vi "App - analyze RUS V6.vi"() -> ()   [LabVIEW 2018] (continued)
__130814c/5_Cooling_2nd_try/September_2014/091714/83.49500K_500_2500_2.10000V_0.00000T_Sep17-2014__00-50-47_001_091714.bin", "last mod"=timestamp(3493774247 s since 1904-01-01), "file name str"="D:\\Data\\Ultrasound\\LSCO\\LSCO22__130814c\\5_Cooling_2nd_try\\September_2014\\091714\\83.49500K_500_2500_2.10000V_0.00000T_Sep17-2014__00-50-47_001_091714.bin", "mod time(min)"=58229570.78333333, "file format"=enum."binary", "power(V)"=2.1, "Magn Field(T) "=0.0}, {"temperature"=83.396, "temperature str"="83.39600", "file path"=path "D:/Data/Ultrasound/LSCO/LSCO22__130814c/5_Cooling_2nd_try/September_2014/091714/83.39600K_500_2500_2.10000V_0.00000T_Sep17-2014__00-52-06_001_091714.bin", "last mod"=timestamp(3493774326 s since 1904-01-01), "file name str"="D:\\Data\\Ultrasound\\LSCO\\LSCO22__130814c\\5_Cooling_2nd_try\\September_2014\\091714\\83.39600K_500_2500_2.10000V_0.00000T_Sep17-2014__00-52-06_001_091714.bin", "mod time(min)"=58229572.1, "file format"=enum."binary", "power(V)"=2.1, "Magn Field(T) "=0.0}, {"temperature"=83.298, "temperature str"="83.29800", "file path"=path "D:/Data/Ultrasound/LSCO/LSCO22__130814c/5_Cooling_2nd_try/September_2014/091714/83.29800K_500_2500_2.10000V_0.00000T_Sep17-2014__00-53-26_001_091714.bin", "last mod"=timestamp(3493774406 s since 1904-01-01), "file name str"="D:\\Data\\Ultrasound\\LSCO\\LSCO22__130814c\\5_Cooling_2nd_try\\September_2014\\091714\\83.29800K_500_2500_2.10000V_0.00000T_Sep17-2014__00-53-26_001_091714.bin", "mod time(min)"=58229573.43333333, "file format"=enum."binary", "power(V)"=2.1, "Magn Field(T) "=0.0}, {"temperature"=83.202, "temperature str"="83.20200", "file path"=path "D:/Data/Ultrasound/LSCO/LSCO22__130814c/5_Cooling_2nd_try/September_2014/091714/83.20200K_500_2500_2.10000V_0.00000T_Sep17-2014__00-54-45_001_091714.bin", "last mod"=timestamp(3493774485 s since 1904-01-01), "file name str"="D:\\Data\\Ultrasound\\LSCO\\LSCO22__130814c\\5_Cooling_2nd_try\\September_2014\\091714\\83.20200K_500_2500_2.10000V_0.00000T_Sep17-2014__00-54-45_001_091714.bin", "mod time(min)"=58229574.75, "file format"=enum."binary", "power(V)"=2.1, "Magn Field(T) "=0.0}, {"temperature"=83.102, "temperature str"="83.10200", "file path"=path "D:/Data/Ultrasound/LSCO/LSCO22__130814c/5_Cooling_2nd_try/September_2014/091714/83.10200K_500_2500_2.10000V_0.00000T_Sep17-2014__00-56-04_001_091714.bin", "last mod"=timestamp(3493774564 s since 1904-01-01), "file name str"="D:\\Data\\Ultrasound\\LSCO\\LSCO22__130814c\\5_Cooling_2nd_try\\September_2014\\091714\\83.10200K_500_2500_2.10000V_0.00000T_Sep17-2014__00-56-04_001_091714.bin", "mod time(min)"=58229576.06666667, "file format"=enum."binary", "power(V)"=2.1, "Magn Field(T) "=0.0}, {"temperature"=83.008, "temperature str"="83.00800", "file path"=path "D:/Data/Ultrasound/LSCO/LSCO22__130814c/5_Cooling_2nd_try/September_2014/091714/83.00800K_500_2500_2.10000V_0.00000T_Sep17-2014__00-57-24_001_091714.bin", "last mod"=timestamp(3493774644 s since 1904-01-01), "file name str"="D:\\Data\\Ultrasound\\LSCO\\LSCO22__130814c\\5_Cooling_2nd_try\\September_2014\\091714\\83.00800K_500_2500_2.10000V_0.00000T_Sep17-2014__00-57-24_001_091714.bin", "mod time(min)"=58229577.4, "file format"=enum."binary", "power(V)"=2.1, "Magn Field(T) "=0.0}, {"temperature"=82.91, "temperature str"="82.91000", "file path"=path "D:/Data/Ultrasound/LSCO/LSCO22__130814c/5_Cooling_2nd_try/September_2014/091714/82.91000K_500_2500_2.10000V_0.00000T_Sep17-2014__00-58-43_001_091714.bin", "last mod"=timestamp(3493774723 s since 1904-01-01), "file name str"="D:\\Data\\Ultrasound\\LSCO\\LSCO22__130814c\\5_Cooling_2nd_try\\September_2014\\091714\\82.91000K_500_2500_2.10000V_0.00000T_Sep17-2014__00-58-43_001_091714.bin", "mod time(min)"=58229578.71666667, "file format"=enum."binary", "power(V)"=2.1, "Magn Field(T) "=0.0}, {"temperature"=82.813, "temperature str"="82.81300", "file path"=path "D:/Data/Ultrasound/LSCO/LSCO22__130814c/5_Cooling_2nd_try/September_2014/091714/82.81300K_500_2500_2.10000V_0.00000T_Sep17-2014__01-00-03_001_091714.bin", "last mod"=timestamp(3493774803 s since 1904-01-01), "file name str"="D:\\Data\\Ultrasound\\LSCO\\LSCO22__130814c\\5_Cooling_2nd_try\\September_2014\\091714\\82.81300K_500_2500_2.10000V_0.00000T_Sep17-2014__01-00-03_001_091714.bin", "mod time(min)"=58229580.05, "file format"=enum."binary", "power(V)"=2.1, "Magn Field(T) "=0.0}, {"temperature"=82.719, "temperature str"="82.71900", "file path"=path "D:/Data/Ultrasound/LSCO/LSCO22__130814c/5_Cooling_2nd_try/September_2014/091714/82.71900K_500_2500_2.10000V_0.00000T_Sep17-2014__01-01-22_001_091714.bin", "last mod"=timestamp(3493774882 s since 1904-01-01), "file name str"="D:\\Data\\Ultrasound\\LSCO\\LSCO22__130814c\\5_Cooling_2nd_try\\September_2014\\091714\\82.71900K_500_2500_2.10000V_0.00000T_Sep17-2014__01-01-22_001_091714.bin", "mod time(min)"=58229581.36666667, "file format"=enum."binary", "power(V)"=2.1, "Magn Field(T) "=0.0}, {"temperature"=82.621, "temperature str"="82.62100", "file path"=path "D:/Data/Ultrasound/LSCO/LSCO22__130814c/5_Cooling_2nd_try/September_2014/091714/82.62100K_500_2500_2.10000V_0.00000T_Sep17-2014__01-02-41_001_091714.bin", "last mod"=timestamp(3493774961 s since 1904-01-01), "file name str"="D:\\Data\\Ultrasound\\LSCO\\LSCO22__130814c\\5_Cooling_2nd_try\\September_2014\\091714\\82.62100K_500_2500_2.10000V_0.00000T_Sep17-2014__01-02-41_001_091714.bin", "mod time(min)"=58229582.68333333, "file format"=enum."binary", "power(V)"=2.1, "Magn Field(T) "=0.0}, {"temperature"=82.529, "temperature str"="82.52900", "file path"=path "D:/Data/Ultrasound/LSCO/LSCO22__130814c/5_Cooling_2nd_try/September_2014/091714/82.52900K_500_2500_2.10000V_0.00000T_Sep17-2014__01-04-01_001_091714.bin", "last mod"=timestamp(3493775041 s since 1904-01-01), "file name str"="D:\\Data\\Ultrasound\\LSCO\\LSCO22__130814c\\5_Cooling_2nd_try\\September_2014\\091714\\82.52900K_500_2500_2.10000V_0.00000T_Sep17-2014__01-04-01_001_091714.bin", "mod time(min)"=58229584.016666666, "file format"=enum."binary", "power(V)"=2.1, "Magn Field(T) "=0.0}, {"temperature"=82.431, "temperature str"="82.43100", "file path"=path "D:/Data/Ultrasound/LSCO/LSCO22__130814c/5_Cooling_2nd_try/September_2014/091714/82.43100K_500_2500_2.10000V_0.00000T_Sep17-2014__01-05-20_001_091714.bin", "last mod"=timestamp(3493775120 s since 1904-01-01), "file name str"="D:\\Data\\Ultrasound\\LSCO\\LSCO22__130814c\\5_Cooling_2nd_try\\September_2014\\091714\\82.43100K_500_2500_2.10000V_0.00000T_Sep17-2014__01-05-20_001_091714.bin", "mod time(min)"=58229585.333333336, "file format"=enum."binary", "power(V)"=2.1, "Magn Field(T) "=0.0}, {"temperature"=82.336, "temperature str"="82.33600", "file path"=path "D:/Data/Ultrasound/LSCO/LSCO22__130814c/5_Cooling_2nd_try/September_2014/091714/82.33600K_500_2500_2.10000V_0.00000T_Sep17-2014__01-06-40_001_091714.bin", "last mod"=timestamp(3493775200 s since 1904-01-01), "file name str"="D:\\Data\\Ultrasound\\LSCO\\LSCO22__130814c\\5_Cooling_2nd_try\\September_2014\\091714\\82.33600K_500_2500_2.10000V_0.00000T_Sep17-2014__01-06-40_001_091714.bin", "mod time(min)"=58229586.666666664, "file format"=enum."binary", "power(V)"=2.1, "Magn Field(T) "=0.0}, {"temperature"=82.244, "temperature str"="82.24400", "file path"=path "D:/Data/Ultrasound/LSCO/LSCO22__130814c/5_Cooling_2nd_try/September_2014/091714/82.24400K_500_2500_2.10000V_0.00000T_Sep17-2014__01-07-59_001_091714.bin", "last mod"=timestamp(3493775279 s since 1904-01-01), "file name str"="D:\\Data\\Ultrasound\\LSCO\\LSCO22__130814c\\5_Cooling_2nd_try\\September_2014\\091714\\82.24400K_500_2500_2.10000V_0.00000T_Sep17-2014__01-07-59_001_091714.bin", "mod time(min)"=58229587.983333334, "file format"=enum."binary", "power(V)"=2.1, "Magn Field(T) "=0.0}, {"temperature"=82.149, "temperature str"="82.14900", "file path"=path "D:/Data/Ultrasound/LSCO/LSCO22__130814c/5_Cooling_2nd_try/September_2014/091714/82.14900K_500_2500_2.10000V_0.00000T_Sep17-2014__01-09-19_001_091714.bin", "last mod"=timestamp(3493775359 s since 1904-01-01), "file name str"="D:\\Data\\Ultrasound\\LSCO\\LSCO22__130814c\\5_Cooling_2nd_try\\September_2014\\091714\\82.14900K_500_2500_2.10000V_0.00000T_Sep17-2014__01-09-19_001_091714.bin", "mod time(min)"=58229589.31666667, "file format"=enum."binary", "power(V)"=2.1, "Magn Field(T) "=0.0}, {"temperature"=82.054, "temperature str"="82.05400", "file path"=path "D:/Data/Ultrasound/LSCO/LSCO22__130814c/5_Cooling_2nd_try/September_2014/091714/82.05400K_500_2500_2.10000V_0.00000T_Sep17-2014__01-10-38_001_091714.bin", "last mod"=timestamp(3493775438 s since 1904-01-01), "file name str"="D:\\Data\\Ultrasound\\LSCO\\LSCO22__130814c\\5_Cooling_2nd_try\\September_2014\\091714\\82.05400K_500_2500_2.10000V_0.00000T_Sep17-2014__01-10-38_001_091714.bin", "mod time(min)"=58229590.63333333, "file format"=enum."binary", "power(V)"=2.1, "Magn Field(T) "=0.0}, {"temperature"=81.963, "temperature str"="81.96300", "file path"=path "D:/Data/Ultrasound/LSCO/LSCO22__130814c/5_Cooling_2nd_try/September_2014/091714/81.96300K_500_2500_2.10000V_0.00000T_Sep17-2014__01-11-58_001_091714.bin", "last mod"=timestamp(3493775518 s since 1904-01-01), "file name str"="D:\\Data\\Ultrasound\\LSCO\\LSCO22__130814c\\5_Cooling_2nd_try\\September_2014\\091714\\81.96300K_500_2500_2.10000V_0.00000T_Sep17-2014__01-11-58_001_091714.bin", "mod time(min)"=58229591.96666667, "file format"=enum."binary", "power(V)"=2.1, "Magn Field(T) "=0.0}, {"temperature"=81.869, "temperature str"="81.86900", "file path"=path "D:/Data/Ultrasound/LSCO/LSCO22__130814c/5_Cooling_2nd_try/September_2014/091714/81.86900K_500_2500_2.10000V_0.00000T_Sep17-2014__01-13-17_001_091714.bin", "last mod"=timestamp(3493775597 s since 1904-01-01), "file name str"="D:\\Data\\Ultrasound\\LSCO\\LSCO22__130814c\\5_Cooling_2nd_try\\September_2014\\091714\\81.86900K_500_2500_2.10000V_0.00000T_Sep17-2014__01-13-17_001_091714.bin", "mod time(min)"=58229593.28333333, "file format"=enum."binary", "power(V)"=2.1, "Magn Field(T) "=0.0}, {"temperature"=81.779, "temperature str"="81.77900", "file path"=path "D:/Data/Ultrasound/LSCO/LSCO22__130814c/5_Cooling_2nd_try/September_2014/091714/81.77900K_500_2500_2.10000V_0.00000T_Sep17-2014__01-14-37_001_091714.bin", "last mod"=timestamp(3493775677 s since 1904-01-01), "file name str"="D:\\Data\\Ultrasound\\LSCO\\LSCO22__130814c\\5_Cooling_2nd_try\\September_2014\\091714\\81.77900K_500_2500_2.10000V_0.00000T_Sep17-2014__01-14-37_001_091714.bin", "mod time(min)"=58229594.61666667, "file format"=enum."binary", "power(V)"=2.1, "Magn Field(T) "=0.0}, {"temperature"=81.683, "temperature str"="81.68300", "file path"=path "D:/Data/Ultrasound/LSCO/LSCO22__130814c/5_Cooling_2nd_try/September_2014/091714/81.68300K_500_2500_2.10000V_0.00000T_Sep17-2014__01-15-56_001_091714.bin", "last mod"=timestamp(3493775756 s since 1904-01-01), "file name str"="D:\\Data\\Ultrasound\\LSCO\\LSCO22__130814c\\5_Cooling_2nd_try\\September_2014\\091714\\81.68300K_500_2500_2.10000V_0.00000T_Sep17-2014__01-15-56_001_091714.bin", "mod time(min)"=58229595.93333333, "file format"=enum."binary", "power(V)"=2.1, "Magn Field(T) "=0.0}, {"temperature"=81.594, "temperature str"="81.59400", "file path"=path "D:/Data/Ultrasound/LSCO/LSCO22__130814c/5_Cooling_2nd_try/September_2014/091714/81.59400K_500_2500_2.10000V_0.00000T_Sep17-2014__01-17-15_001_091714.bin", "last mod"=timestamp(3493775835 s since 1904-01-01), "file name str"="D:\\Data\\Ultrasound\\LSCO\\LSCO22__130814c\\5_Cooling_2nd_try\\September_2014\\091714\\81.59400K_500_2500_2.10000V_0.00000T_Sep17-2014__01-17-15_001_091714.bin", "mod time(min)"=58229597.25, "file format"=enum."binary", "power(V)"=2.1, "Magn Field(T) "=0.0}, {"temperature"=81.501, "temperature str"="81.50100", "file path"=path "D:/Data/Ultrasound/LSCO/LSCO22__130814c/5_Cooling_2nd_try/September_2014/091714/81.50100K_500_2500_2.10000V_0.00000T_Sep17-2014__01-18-35_001_091714.bin", "last mod"=timestamp(3493775915 s since 1904-01-01), "file name str"="D:\\Data\\Ultrasound\\LSCO\\LSCO22__130814c\\5_Cooling_2nd_try\\September_2014\\091714\\81.50100K_500_2500_2.10000V_0.00000T_Sep17-2014__01-18-35_001_091714.bin", "mod time(min)"=58229598.583333336, "file format"=enum."binary", "power(V)"=2.1, "Magn Field(T) "=0.0}, {"temperature"=81.408, "temperature str"="81.40800", "file path"=path "D:/Data/Ultrasound/LSCO/LSCO22__130814c/5_Cooling_2nd_try/September_2014/091714/81.40800K_500_2500_2.10000V_0.00000T_Sep17-2014__01-19-54_001_091714.bin", "last mod"=timestamp(3493775994 s since 1904-01-01), "file name str"="D:\\Data\\Ultrasound\\LSCO\\LSCO22__130814c\\5_Cooling_2nd_try\\September_2014\\091714\\81.40800K_500_2500_2.10000V_0.00000T_Sep17-2014__01-19-54_001_091714.bin", "mod time(min)"=58229599.9, "file format"=enum."binary", "power(V)"=2.1, "Magn Field(T) "=0.0}, {"temperature"=81.32, "temperature str"="81.32000", "file path"=path "D:/Data/Ultrasound/LSCO/LSCO22__130814c/5_Cooling_2nd_try/September_2014/091714/81.32000K_500_2500_2.10000V_0.00000T_Sep17-2014__01-21-13_001_091714.bin", "last mod"=timestamp(3493776073 s since 1904-01-01), "file name str"="D:\\Data\\Ultrasound\\LSCO\\LSCO22__130814c\\5_Cooling_2nd_try\\September_2014\\091714\\81.32000K_500_2500_2.10000V_0.00000T_Sep17-2014__01-21-13_001_091714.bin", "mod time(min)"=58229601.21666667, "file format"=enum."binary", "power(V)"=2.1, "Magn Field(T) "=0.0}, {"temperature"=81.229, "temperature str"="81.22900", "file path"=path "D:/Data/Ultrasound/LSCO/LSCO22__130814c/5_Cooling_2nd_try/September_2014/091714/81.22900K_500_2500_2.10000V_0.00000T_Sep17-2014__01-22-33_001_091714.bin", "last mod"=timestamp(3493776153 s since 1904-01-01), "file name str"="D:\\Data\\Ultrasound\\LSCO\\LSCO22__130814c\\5_Cooling_2nd_try\\September_2014\\091714\\81.22900K_500_2500_2.10000V_0.00000T_Sep17-2014__01-22-33_001_091714.bin", "mod time(min)"=58229602.55, "file format"=enum."binary", "power(V)"=2.1, "Magn Field(T) "=0.0}, {"temperature"=81.134, "temperature str"="81.13400", "file path"=path "D:/Data/Ultrasound/LSCO/LSCO22__130814c/5_Cooling_2nd_try/September_2014/091714/81.13400K_500_2500_2.10000V_0.00000T_Sep17-2014__01-23-52_001_091714.bin", "last mod"=timestamp(3493776232 s since 1904-01-01), "file name str"="D:\\Data\\Ultrasound\\LSCO\\LSCO22__130814c\\5_Cooling_2nd_try\\September_2014\\091714\\81.13400K_500_2500_2.10000V_0.00000T_Sep17-2014__01-23-52_001_091714.bin", "mod time(min)"=58229603.86666667, "file format"=enum."binary", "power(V)"=2.1, "Magn Field(T) "=0.0}, {"temperature"=81.047, "temperature str"="81.04700", "file path"=path "D:/Data/Ultrasound/LSCO/LSCO22__130814c/5_Cooling_2nd_try/September_2014/091714/81.04700K_500_2500_2.10000V_0.00000T_Sep17-2014__01-25-12_001_091714.bin", "last mod"=timestamp(3493776312 s since 1904-01-01), "file name str"="D:\\Data\\Ultrasound\\LSCO\\LSCO22__130814c\\5_Cooling_2nd_try\\September_2014\\091714\\81.04700K_500_2500_2.10000V_0.00000T_Sep17-2014__01-25-12_001_091714.bin", "mod time(min)"=58229605.2, "file format"=enum."binary", "power(V)"=2.1, "Magn Field(T) "=0.0}, {"temperature"=80.958, "temperature str"="80.95800", "file path"=path "D:/Data/Ultrasound/LSCO/LSCO22__130814c/5_Cooling_2nd_try/September_2014/091714/80.95800K_500_2500_2.10000V_0.00000T_Sep17-2014__01-26-31_001_091714.bin", "last mod"=timestamp(3493776391 s since 1904-01-01), "file name str"="D:\\Data\\Ultrasound\\LSCO\\LSCO22__130814c\\5_Cooling_2nd_try\\September_2014\\091714\\80.95800K_500_2500_2.10000V_0.00000T_Sep17-2014__01-26-31_001_091714.bin", "mod time(min)"=58229606.516666666, "file format"=enum."binary", "power(V)"=2.1, "Magn Field(T) "=0.0}, {"temperature"=80.871, "temperature str"="80.87100", "file path"=path "D:/Data/Ultrasound/LSCO/LSCO22__130814c/5_Cooling_2nd_try/September_2014/091714/80.87100K_500_2500_2.10000V_0.00000T_Sep17-2014__01-27-50_001_091714.bin", "last mod"=timestamp(3493776470 s since 1904-01-01), "file name str"="D:\\Data\\Ultrasound\\LSCO\\LSCO22__130814c\\5_Cooling_2nd_try\\September_2014\\091714\\80.87100K_500_2500_2.10000V_0.00000T_Sep17-2014__01-27-50_001_091714.bin", "mod time(min)"=58229607.833333336, "file format"=enum."binary", "power(V)"=2.1, "Magn Field(T) "=0.0}, {"temperature"=80.778, "temperature str"="80.77800", "file path"=path "D:/Data/Ultrasound/LSCO/LSCO22__130814c/5_Cooling_2nd_try/September_2014/091714/80.77800K_500_2500_2.10000V_0.00000T_Sep17-2014__01-29-10_001_091714.bin", "last mod"=timestamp(3493776550 s since 1904-01-01), "file name str"="D:\\Data\\Ultrasound\\LSCO\\LSCO22__130814c\\5_Cooling_2nd_try\\September_2014\\091714\\80.77800K_500_2500_2.10000V_0.00000T_Sep17-2014__01-29-10_001_091714.bin", "mod time(min)"=58229609.166666664, "file format"=enum."binary", "power(V)"=2.1, "Magn Field(T) "=0.0}, {"temperature"=80.688, "temperature str"="80.68800", "file path"=path "D:/Data/Ultrasound/LSCO/LSCO22__130814c/5_Cooling_2nd_try/September_2014/091714/80.68800K_500_2500_2.10000V_0.00000T_Sep17-2014__01-30-29_001_091714.bin", "last mod"=timestamp(3493776629 s since 1904-01-01), "file name str"="D:\\Data\\Ultrasound\\LSCO\\LSCO22__130814c\\5_Cooling_2nd_try\\September_2014\\091714\\80.68800K_500_2500_2.10000V_0.00000T_Sep17-2014__01-30-29_001_091714.bin", "mod time(min)"=58229610.483333334, "file format"=enum."binary", "power(V)"=2.1, "Magn Field(T) "=0.0}, {"temperature"=80.602, "temperature str"="80.60200", "file path"=path "D:/Data/Ultrasound/LSCO/LSCO22__130814c/5_Cooling_2nd_try/September_2014/091714/80.60200K_500_2500_2.10000V_0.00000T_Sep17-2014__01-31-49_001_091714.bin", "last mod"=timestamp(3493776709 s since 1904-01-01), "file name str"="D:\\Data\\Ultrasound\\LSCO\\LSCO22__130814c\\5_Cooling_2nd_try\\September_2014\\091714\\80.60200K_500_2500_2.10000V_0.00000T_Sep17-2014__01-31-49_001_091714.bin", "mod time(min)"=58229611.81666667, "file format"=enum."binary", "power(V)"=2.1, "Magn Field(T) "=0.0}, {"temperature"=80.512, "temperature str"="80.51200", "file path"=path "D:/Data/Ultrasound/LSCO/LSCO22__130814c/5_Cooling_2nd_try/September_2014/091714/80.51200K_500_2500_2.10000V_0.00000T_Sep17-2014__01-33-08_001_091714.bin", "last mod"=timestamp(3493776788 s since 1904-01-01), "file name str"="D:\\Data\\Ultrasound\\LSCO\\LSCO22__130814c\\5_Cooling_2nd_try\\September_2014\\091714\\80.51200K_500_2500_2.10000V_0.00000T_Sep17-2014__01-33-08_001_091714.bin", "mod time(min)"=58229613.13333333, "file format"=enum."binary", "power(V)"=2.1, "Magn Field(T) "=0.0}, {"temperature"=80.428, "temperature str"="80.42800", "file path"=path "D:/Data/Ultrasound/LSCO/LSCO22__130814c/5_Cooling_2nd_try/September_2014/091714/80.42800K_500_2500_2.10000V_0.00000T_Sep17-2014__01-34-27_001_091714.bin", "last mod"=timestamp(3493776867 s since 1904-01-01), "file name str"="D:\\Data\\Ultrasound\\LSCO\\LSCO22__130814c\\5_Cooling_2nd_try\\September_2014\\091714\\80.42800K_500_2500_2.10000V_0.00000T_Sep17-2014__01-34-27_001_091714.bin", "mod time(min)"=58229614.45, "file format"=enum."binary", "power(V)"=2.1, "Magn Field(T) "=0.0}, {"temperature"=80.338, "temperature str"="80.33800", "file path"=path "D:/Data/Ultrasound/LSCO/LSCO22__130814c/5_Cooling_2nd_try/September_2014/091714/80.33800K_500_2500_2.10000V_0.00000T_Sep17-2014__01-35-47_001_091714.bin", "last mod"=timestamp(3493776947 s since 1904-01-01), "file name str"="D:\\Data\\Ultrasound\\LSCO\\LSCO22__130814c\\5_Cooling_2nd_try\\September_2014\\091714\\80.33800K_500_2500_2.10000V_0.00000T_Sep17-2014__01-35-47_001_091714.bin", "mod time(min)"=58229615.78333333, "file format"=enum."binary", "power(V)"=2.1, "Magn Field(T) "=0.0}, {"temperature"=80.249, "temperature str"="80.24900", "file path"=path "D:/Data/Ultrasound/LSCO/LSCO22__130814c/5_Cooling_2nd_try/September_2014/091714/80.24900K_500_2500_2.10000V_0.00000T_Sep17-2014__01-37-06_001_091714.bin", "last mod"=timestamp(3493777026 s since 1904-01-01), "file name str"="D:\\Data\\Ultrasound\\LSCO\\LSCO22__130814c\\5_Cooling_2nd_try\\September_2014\\091714\\80.24900K_500_2500_2.10000V_0.00000T_Sep17-2014__01-37-06_001_091714.bin", "mod time(min)"=58229617.1, "file format"=enum."binary", "power(V)"=2.1, "Magn Field(T) "=0.0}, {"temperature"=80.163, "temperature str"="80.16300", "file path"=path "D:/Data/Ultrasound/LSCO/LSCO22__130814c/5_Cooling_2nd_try/September_2014/091714/80.16300K_500_2500_2.10000V_0.00000T_Sep17-2014__01-38-25_001_091714.bin", "last mod"=timestamp(3493777105 s since 1904-01-01), "file name str"="D:\\Data\\Ultrasound\\LSCO\\LSCO22__130814c\\5_Cooling_2nd_try\\September_2014\\091714\\80.16300K_500_2500_2.10000V_0.00000T_Sep17-2014__01-38-25_001_091714.bin", "mod time(min)"=58229618.416666664, "file format"=enum."binary", "power(V)"=2.1, "Magn Field(T) "=0.0}, {"temperature"=80.075, "temperature str"="80.07500", "file path"=path "D:/Data/Ultrasound/LSCO/LSCO22__130814c/5_Cooling_2nd_try/September_2014/091714/80.07500K_500_2500_2.10000V_0.00000T_Sep17-2014__01-39-45_001_091714.bin", "last mod"=timestamp(3493777185 s since 1904-01-01), "file name str"="D:\\Data\\Ultrasound\\LSCO\\LSCO22__130814c\\5_Cooling_2nd_try\\September_2014\\091714\\80.07500K_500_2500_2.10000V_0.00000T_Sep17-2014__01-39-45_001_091714.bin", "mod time(min)"=58229619.75, "file format"=enum."binary", "power(V)"=2.1, "Magn Field(T) "=0.0}, {"temperature"=79.991, "temperature str"="79.99100", "file path"=path "D:/Data/Ultrasound/LSCO/LSCO22__130814c/5_Cooling_2nd_try/September_2014/091714/79.99100K_500_2500_2.10000V_0.00000T_Sep17-2014__01-41-04_001_091714.bin", "last mod"=timestamp(3493777264 s since 1904-01-01), "file name str"="D:\\Data\\Ultrasound\\LSCO\\LSCO22__130814c\\5_Cooling_2nd_try\\September_2014\\091714\\79.99100K_500_2500_2.10000V_0.00000T_Sep17-2014__01-41-04_001_091714.bin", "mod time(min)"=58229621.06666667, "file format"=enum."binary", "power(V)"=2.1, "Magn Field(T) "=0.0}, {"temperature"=79.903, "temperature str"="79.90300", "file path"=path "D:/Data/Ultrasound/LSCO/LSCO22__130814c/5_Cooling_2nd_try/September_2014/091714/79.90300K_500_2500_2.10000V_0.00000T_Sep17-2014__01-42-24_001_091714.bin", "last mod"=timestamp(3493777344 s since 1904-01-01), "file name str"="D:\\Data\\Ultrasound\\LSCO\\LSCO22__130814c\\5_Cooling_2nd_try\\September_2014\\091714\\79.90300K_500_2500_2.10000V_0.00000T_Sep17-2014__01-42-24_001_091714.bin", "mod time(min)"=58229622.4, "file format"=enum."binary", "power(V)"=2.1, "Magn Field(T) "=0.0}, {"temperature"=79.817, "temperature str"="79.81700", "file path"=path "D:/Data/Ultrasound/LSCO/LSCO22__130814c/5_Cooling_2nd_try/September_2014/091714/79.81700K_500_2500_2.10000V_0.00000T_Sep17-2014__01-43-43_001_091714.bin", "last mod"=timestamp(3493777423 s since 1904-01-01), "file name str"="D:\\Data\\Ultrasound\\LSCO\\LSCO22__130814c\\5_Cooling_2nd_try\\September_2014\\091714\\79.81700K_500_2500_2.10000V_0.00000T_Sep17-2014__01-43-43_001_091714.bin", "mod time(min)"=58229623.71666667, "file format"=enum."binary", "power(V)"=2.1, "Magn Field(T) "=0.0}, {"temperature"=79.734, "temperature str"="79.73400", "file path"=path "D:/Data/Ultrasound/LSCO/LSCO22__130814c/5_Cooling_2nd_try/September_2014/091714/79.73400K_500_2500_2.10000V_0.00000T_Sep17-2014__01-45-02_001_091714.bin", "last mod"=timestamp(3493777502 s since 1904-01-01), "file name str"="D:\\Data\\Ultrasound\\LSCO\\LSCO22__130814c\\5_Cooling_2nd_try\\September_2014\\091714\\79.73400K_500_2500_2.10000V_0.00000T_Sep17-2014__01-45-02_001_091714.bin", "mod time(min)"=58229625.03333333, "file format"=enum."binary", "power(V)"=2.1, "Magn Field(T) "=0.0}, {"temperature"=79.645, "temperature str"="79.64500", "file path"=path "D:/Data/Ultrasound/LSCO/LSCO22__130814c/5_Cooling_2nd_try/September_2014/091714/79.64500K_500_2500_2.10000V_0.00000T_Sep17-2014__01-46-22_001_091714.bin", "last mod"=timestamp(3493777582 s since 1904-01-01), "file name str"="D:\\Data\\Ultrasound\\LSCO\\LSCO22__130814c\\5_Cooling_2nd_try\\September_2014\\091714\\79.64500K_500_2500_2.10000V_0.00000T_Sep17-2014__01-46-22_001_091714.bin", "mod time(min)"=58229626.36666667, "file format"=enum."binary", "power(V)"=2.1, "Magn Field(T) "=0.0}, {"temperature"=79.564, "temperature str"="79.56400", "file path"=path "D:/Data/Ultrasound/LSCO/LSCO22__130814c/5_Cooling_2nd_try/September_2014/091714/79.56400K_500_2500_2.10000V_0.00000T_Sep17-2014__01-47-41_001_091714.bin", "last mod"=timestamp(3493777661 s since 1904-01-01), "file name str"="D:\\Data\\Ultrasound\\LSCO\\LSCO22__130814c\\5_Cooling_2nd_try\\September_2014\\091714\\79.56400K_500_2500_2.10000V_0.00000T_Sep17-2014__01-47-41_001_091714.bin", "mod time(min)"=58229627.68333333, "file format"=enum."binary", "power(V)"=2.1, "Magn Field(T) "=0.0}, {"temperature"=79.476, "temperature str"="79.47600", "file path"=path "D:/Data/Ultrasound/LSCO/LSCO22__130814c/5_Cooling_2nd_try/September_2014/091714/79.47600K_500_2500_2.10000V_0.00000T_Sep17-2014__01-49-00_001_091714.bin", "last mod"=timestamp(3493777740 s since 1904-01-01), "file name str"="D:\\Data\\Ultrasound\\LSCO\\LSCO22__130814c\\5_Cooling_2nd_try\\September_2014\\091714\\79.47600K_500_2500_2.10000V_0.00000T_Sep17-2014__01-49-00_001_091714.bin", "mod time(min)"=58229629.0, "file format"=enum."binary", "power(V)"=2.1, "Magn Field(T) "=0.0}, {"temperature"=79.39, "temperature str"="79.39000", "file path"=path "D:/Data/Ultrasound/LSCO/LSCO22__130814c/5_Cooling_2nd_try/September_2014/091714/79.39000K_500_2500_2.10000V_0.00000T_Sep17-2014__01-50-20_001_091714.bin", "last mod"=timestamp(3493777820 s since 1904-01-01), "file name str"="D:\\Data\\Ultrasound\\LSCO\\LSCO22__130814c\\5_Cooling_2nd_try\\September_2014\\091714\\79.39000K_500_2500_2.10000V_0.00000T_Sep17-2014__01-50-20_001_091714.bin", "mod time(min)"=58229630.333333336, "file format"=enum."binary", "power(V)"=2.1, "Magn Field(T) "=0.0}, {"temperature"=79.307, "temperature str"="79.30700", "file path"=path "D:/Data/Ultrasound/LSCO/LSCO22__130814c/5_Cooling_2nd_try/September_2014/091714/79.30700K_500_2500_2.10000V_0.00000T_Sep17-2014__01-51-39_001_091714.bin", "last mod"=timestamp(3493777899 s since 1904-01-01), "file name str"="D:\\Data\\Ultrasound\\LSCO\\LSCO22__130814c\\5_Cooling_2nd_try\\September_2014\\091714\\79.30700K_500_2500_2.10000V_0.00000T_Sep17-2014__01-51-39_001_091714.bin", "mod time(min)"=58229631.65, "file format"=enum."binary", "power(V)"=2.1, "Magn Field(T) "=0.0}, {"temperature"=79.224, "temperature str"="79.22400", "file path"=path "D:/Data/Ultrasound/LSCO/LSCO22__130814c/5_Cooling_2nd_try/September_2014/091714/79.22400K_500_2500_2.10000V_0.00000T_Sep17-2014__01-52-59_001_091714.bin", "last mod"=timestamp(3493777979 s since 1904-01-01), "file name str"="D:\\Data\\Ultrasound\\LSCO\\LSCO22__130814c\\5_Cooling_2nd_try\\September_2014\\091714\\79.22400K_500_2500_2.10000V_0.00000T_Sep17-2014__01-52-59_001_091714.bin", "mod time(min)"=58229632.983333334, "file format"=enum."binary", "power(V)"=2.1, "Magn Field(T) "=0.0}, {"temperature"=79.141, "temperature str"="79.14100", "file path"=path "D:/Data/Ultrasound/LSCO/LSCO22__130814c/5_Cooling_2nd_try/September_2014/091714/79.14100K_500_2500_2.10000V_0.00000T_Sep17-2014__01-54-18_001_091714.bin", "last mod"=timestamp(3493778058 s since 1904-01-01), "file name str"="D:\\Data\\Ultrasound\\LSCO\\LSCO22__130814c\\5_Cooling_2nd_try\\September_2014\\091714\\79.14100K_500_2500_2.10000V_0.00000T_Sep17-2014__01-54-18_001_091714.bin", "mod time(min)"=58229634.3, "file format"=enum."binary", "power(V)"=2.1, "Magn Field(T) "=0.0}, {"temperature"=79.055, "temperature str"="79.05500", "file path"=path "D:/Data/Ultrasound/LSCO/LSCO22__130814c/5_Cooling_2nd_try/September_2014/091714/79.05500K_500_2500_2.10000V_0.00000T_Sep17-2014__01-55-37_001_091714.bin", "last mod"=timestamp(3493778137 s since 1904-01-01), "file name str"="D:\\Data\\Ultrasound\\LSCO\\LSCO22__130814c\\5_Cooling_2nd_try\\September_2014\\091714\\79.05500K_500_2500_2.10000V_0.00000T_Sep17-2014__01-55-37_001_091714.bin", "mod time(min)"=58229635.61666667, "file format"=enum."binary", "power(V)"=2.1, "Magn Field(T) "=0.0}, {"temperature"=78.972, "temperature str"="78.97200", "file path"=path "D:/Data/Ultrasound/LSCO/LSCO22__130814c/5_Cooling_2nd_try/September_2014/091714/78.97200K_500_2500_2.10000V_0.00000T_Sep17-2014__01-56-57_001_091714.bin", "last mod"=timestamp(3493778217 s since 1904-01-01), "file name str"="D:\\Data\\Ultrasound\\LSCO\\LSCO22__130814c\\5_Cooling_2nd_try\\September_2014\\091714\\78.97200K_500_2500_2.10000V_0.00000T_Sep17-2014__01-56-57_001_091714.bin", "mod time(min)"=58229636.95, "file format"=enum."binary", "power(V)"=2.1, "Magn Field(T) "=0.0}, {"temperature"=78.889, "temperature str"="78.88900", "file path"=path "D:/Data/Ultrasound/LSCO/LSCO22__130814c/5_Cooling_2nd_try/September_2014/091714/78.88900K_500_2500_2.10000V_0.00000T_Sep17-2014__01-58-16_001_091714.bin", "last mod"=timestamp(3493778296 s since 1904-01-01), "file name str"="D:\\Data\\Ultrasound\\LSCO\\LSCO22__130814c\\5_Cooling_2nd_try\\September_2014\\091714\\78.88900K_500_2500_2.10000V_0.00000T_Sep17-2014__01-58-16_001_091714.bin", "mod time(min)"=58229638.266666666, "file format"=enum."binary", "power(V)"=2.1, "Magn Field(T) "=0.0}, {"temperature"=78.806, "temperature str"="78.80600", "file path"=path "D:/Data/Ultrasound/LSCO/LSCO22__130814c/5_Cooling_2nd_try/September_2014/091714/78.80600K_500_2500_2.10000V_0.00000T_Sep17-2014__01-59-35_001_091714.bin", "last mod"=timestamp(3493778375 s since 1904-01-01), "file name str"="D:\\Data\\Ultrasound\\LSCO\\LSCO22__130814c\\5_Cooling_2nd_try\\September_2014\\091714\\78.80600K_500_2500_2.10000V_0.00000T_Sep17-2014__01-59-35_001_091714.bin", "mod time(min)"=58229639.583333336, "file format"=enum."binary", "power(V)"=2.1, "Magn Field(T) "=0.0}, {"temperature"=78.721, "temperature str"="78.72100", "file path"=path "D:/Data/Ultrasound/LSCO/LSCO22__130814c/5_Cooling_2nd_try/September_2014/091714/78.72100K_500_2500_2.10000V_0.00000T_Sep17-2014__02-00-55_001_091714.bin", "last mod"=timestamp(3493778455 s since 1904-01-01), "file name str"="D:\\Data\\Ultrasound\\LSCO\\LSCO22__130814c\\5_Cooling_2nd_try\\September_2014\\091714\\78.72100K_500_2500_2.10000V_0.00000T_Sep17-2014__02-00-55_001_091714.bin", "mod time(min)"=58229640.916666664, "file format"=enum."binary", "power(V)"=2.1, "Magn Field(T) "=0.0}, {"temperature"=78.641, "temperature str"="78.64100", "file path"=path "D:/Data/Ultrasound/LSCO/LSCO22__130814c/5_Cooling_2nd_try/September_2014/091714/78.64100K_500_2500_2.10000V_0.00000T_Sep17-2014__02-02-14_001_091714.bin", "last mod"=timestamp(3493778534 s since 1904-01-01), "file name str"="D:\\Data\\Ultrasound\\LSCO\\LSCO22__130814c\\5_Cooling_2nd_try\\September_2014\\091714\\78.64100K_500_2500_2.10000V_0.00000T_Sep17-2014__02-02-14_001_091714.bin", "mod time(min)"=58229642.233333334, "file format"=enum."binary", "power(V)"=2.1, "Magn Field(T) "=0.0}, {"temperature"=78.559, "temperature str"="78.55900", "file path"=path "D:/Data/Ultrasound/LSCO/LSCO22__130814c/5_Cooling_2nd_try/September_2014/091714/78.55900K_500_2500_2.10000V_0.00000T_Sep17-2014__02-03-34_001_091714.bin", "last mod"=timestamp(3493778614 s since 1904-01-01), "file name str"="D:\\Data\\Ultrasound\\LSCO\\LSCO22__130814c\\5_Cooling_2nd_try\\September_2014\\091714\\78.55900K_500_2500_2.10000V_0.00000T_Sep17-2014__02-03-34_001_091714.bin", "mod time(min)"=58229643.56666667, "file format"=enum."binary", "power(V)"=2.1, "Magn Field(T) "=0.0}, {"temperature"=78.479, "temperature str"="78.47900", "file path"=path "D:/Data/Ultrasound/LSCO/LSCO22__130814c/5_Cooling_2nd_try/September_2014/091714/78.47900K_500_2500_2.10000V_0.00000T_Sep17-2014__02-04-53_001_091714.bin", "last mod"=timestamp(3493778693 s since 1904-01-01), "file name str"="D:\\Data\\Ultrasound\\LSCO\\LSCO22__130814c\\5_Cooling_2nd_try\\September_2014\\091714\\78.47900K_500_2500_2.10000V_0.00000T_Sep17-2014__02-04-53_001_091714.bin", "mod time(min)"=58229644.88333333, "file format"=enum."binary", "power(V)"=2.1, "Magn Field(T) "=0.0}, {"temperature"=78.395, "temperature str"="78.39500", "file path"=path "D:/Data/Ultrasound/LSCO/LSCO22__130814c/5_Cooling_2nd_try/September_2014/091714/78.39500K_500_2500_2.10000V_0.00000T_Sep17-2014__02-06-12_001_091714.bin", "last mod"=timestamp(3493778772 s since 1904-01-01), "file name str"="D:\\Data\\Ultrasound\\LSCO\\LSCO22__130814c\\5_Cooling_2nd_try\\September_2014\\091714\\78.39500K_500_2500_2.10000V_0.00000T_Sep17-2014__02-06-12_001_091714.bin", "mod time(min)"=58229646.2, "file format"=enum."binary", "power(V)"=2.1, "Magn Field(T) "=0.0}, {"temperature"=78.313, "temperature str"="78.31300", "file path"=path "D:/Data/Ultrasound/LSCO/LSCO22__130814c/5_Cooling_2nd_try/September_2014/091714/78.31300K_500_2500_2.10000V_0.00000T_Sep17-2014__02-07-32_001_091714.bin", "last mod"=timestamp(3493778852 s since 1904-01-01), "file name str"="D:\\Data\\Ultrasound\\LSCO\\LSCO22__130814c\\5_Cooling_2nd_try\\September_2014\\091714\\78.31300K_500_2500_2.10000V_0.00000T_Sep17-2014__02-07-32_001_091714.bin", "mod time(min)"=58229647.53333333, "file format"=enum."binary", "power(V)"=2.1, "Magn Field(T) "=0.0}, {"temperature"=78.233, "temperature str"="78.23300", "file path"=path "D:/Data/Ultrasound/LSCO/LSCO22__130814c/5_Cooling_2nd_try/September_2014/091714/78.23300K_500_2500_2.10000V_0.00000T_Sep17-2014__02-08-51_001_091714.bin", "last mod"=timestamp(3493778931 s since 1904-01-01), "file name str"="D:\\Data\\Ultrasound\\LSCO\\LSCO22__130814c\\5_Cooling_2nd_try\\September_2014\\091714\\78.23300K_500_2500_2.10000V_0.00000T_Sep17-2014__02-08-51_001_091714.bin", "mod time(min)"=58229648.85, "file format"=enum."binary", "power(V)"=2.1, "Magn Field(T) "=0.0}, {"temperature"=78.151, "temperature str"="78.15100", "file path"=path "D:/Data/Ultrasound/LSCO/LSCO22__130814c/5_Cooling_2nd_try/September_2014/091714/78.15100K_500_2500_2.10000V_0.00000T_Sep17-2014__02-10-11_001_091714.bin", "last mod"=timestamp(3493779011 s since 1904-01-01), "file name str"="D:\\Data\\Ultrasound\\LSCO\\LSCO22__130814c\\5_Cooling_2nd_try\\September_2014\\091714\\78.15100K_500_2500_2.10000V_0.00000T_Sep17-2014__02-10-11_001_091714.bin", "mod time(min)"=58229650.18333333, "file format"=enum."binary", "power(V)"=2.1, "Magn Field(T) "=0.0}, {"temperature"=78.071, "temperature str"="78.07100", "file path"=path "D:/Data/Ultrasound/LSCO/LSCO22__130814c/5_Cooling_2nd_try/September_2014/091714/78.07100K_500_2500_2.10000V_0.00000T_Sep17-2014__02-11-30_001_091714.bin", "last mod"=timestamp(3493779090 s since 1904-01-01), "file name str"="D:\\Data\\Ultrasound\\LSCO\\LSCO22__130814c\\5_Cooling_2nd_try\\September_2014\\091714\\78.07100K_500_2500_2.10000V_0.00000T_Sep17-2014__02-11-30_001_091714.bin", "mod time(min)"=58229651.5, "file format"=enum."binary", "power(V)"=2.1, "Magn Field(T) "=0.0}, {"temperature"=77.989, "temperature str"="77.98900", "file path"=path "D:/Data/Ultrasound/LSCO/LSCO22__130814c/5_Cooling_2nd_try/September_2014/091714/77.98900K_500_2500_2.10000V_0.00000T_Sep17-2014__02-12-49_001_091714.bin", "last mod"=timestamp(3493779169 s since 1904-01-01), "file name str"="D:\\Data\\Ultrasound\\LSCO\\LSCO22__130814c\\5_Cooling_2nd_try\\September_2014\\091714\\77.98900K_500_2500_2.10000V_0.00000T_Sep17-2014__02-12-49_001_091714.bin", "mod time(min)"=58229652.81666667, "file format"=enum."binary", "power(V)"=2.1, "Magn Field(T) "=0.0}, {"temperature"=77.909, "temperature str"="77.90900", "file path"=path "D:/Data/Ultrasound/LSCO/LSCO22__130814c/5_Cooling_2nd_try/September_2014/091714/77.90900K_500_2500_2.10000V_0.00000T_Sep17-2014__02-14-09_001_091714.bin", "last mod"=timestamp(3493779249 s since 1904-01-01), "file name str"="D:\\Data\\Ultrasound\\LSCO\\LSCO22__130814c\\5_Cooling_2nd_try\\September_2014\\091714\\77.90900K_500_2500_2.10000V_0.00000T_Sep17-2014__02-14-09_001_091714.bin", "mod time(min)"=58229654.15, "file format"=enum."binary", "power(V)"=2.1, "Magn Field(T) "=0.0}, {"temperature"=77.83, "temperature str"="77.83000", "file path"=path "D:/Data/Ultrasound/LSCO/LSCO22__130814c/5_Cooling_2nd_try/September_2014/091714/77.83000K_500_2500_2.10000V_0.00000T_Sep17-2014__02-15-28_001_091714.bin", "last mod"=timestamp(3493779328 s since 1904-01-01), "file name str"="D:\\Data\\Ultrasound\\LSCO\\LSCO22__130814c\\5_Cooling_2nd_try\\September_2014\\091714\\77.83000K_500_2500_2.10000V_0.00000T_Sep17-2014__02-15-28_001_091714.bin", "mod time(min)"=58229655.46666667, "file format"=enum."binary", "power(V)"=2.1, "Magn Field(T) "=0.0}, {"temperature"=77.749, "temperature str"="77.74900", "file path"=path "D:/Data/Ultrasound/LSCO/LSCO22__130814c/5_Cooling_2nd_try/September_2014/091714/77.74900K_500_2500_2.10000V_0.00000T_Sep17-2014__02-16-47_001_091714.bin", "last mod"=timestamp(3493779407 s since 1904-01-01), "file name str"="D:\\Data\\Ultrasound\\LSCO\\LSCO22__130814c\\5_Cooling_2nd_try\\September_2014\\091714\\77.74900K_500_2500_2.10000V_0.00000T_Sep17-2014__02-16-47_001_091714.bin", "mod time(min)"=58229656.78333333, "file format"=enum."binary", "power(V)"=2.1, "Magn Field(T) "=0.0}, {"temperature"=77.673, "temperature str"="77.67300", "file path"=path "D:/Data/Ultrasound/LSCO/LSCO22__130814c/5_Cooling_2nd_try/September_2014/091714/77.67300K_500_2500_2.10000V_0.00000T_Sep17-2014__02-18-07_001_091714.bin", "last mod"=timestamp(3493779487 s since 1904-01-01), "file name str"="D:\\Data\\Ultrasound\\LSCO\\LSCO22__130814c\\5_Cooling_2nd_try\\September_2014\\091714\\77.67300K_500_2500_2.10000V_0.00000T_Sep17-2014__02-18-07_001_091714.bin", "mod time(min)"=58229658.11666667, "file format"=enum."binary", "power(V)"=2.1, "Magn Field(T) "=0.0}, {"temperature"=77.593, "temperature str"="77.59300", "file path"=path "D:/Data/Ultrasound/LSCO/LSCO22__130814c/5_Cooling_2nd_try/September_2014/091714/77.59300K_500_2500_2.10000V_0.00000T_Sep17-2014__02-19-26_001_091714.bin", "last mod"=timestamp(3493779566 s since 1904-01-01), "file name str"="D:\\Data\\Ultrasound\\LSCO\\LSCO22__130814c\\5_Cooling_2nd_try\\September_2014\\091714\\77.59300K_500_2500_2.10000V_0.00000T_Sep17-2014__02-19-26_001_091714.bin", "mod time(min)"=58229659.43333333, "file format"=enum."binary", "power(V)"=2.1, "Magn Field(T) "=0.0}, {"temperature"=77.512, "temperature str"="77.51200", "file path"=path "D:/Data/Ultrasound/LSCO/LSCO22__130814c/5_Cooling_2nd_try/September_2014/091714/77.51200K_500_2500_2.10000V_0.00000T_Sep17-2014__02-20-46_001_091714.bin", "last mod"=timestamp(3493779646 s since 1904-01-01), "file name str"="D:\\Data\\Ultrasound\\LSCO\\LSCO22__130814c\\5_Cooling_2nd_try\\September_2014\\091714\\77.51200K_500_2500_2.10000V_0.00000T_Sep17-2014__02-20-46_001_091714.bin", "mod time(min)"=58229660.766666666, "file format"=enum."binary", "power(V)"=2.1, "Magn Field(T) "=0.0}, {"temperature"=77.434, "temperature str"="77.43400", "file path"=path "D:/Data/Ultrasound/LSCO/LSCO22__130814c/5_Cooling_2nd_try/September_2014/091714/77.43400K_500_2500_2.10000V_0.00000T_Sep17-2014__02-22-05_001_091714.bin", "last mod"=timestamp(3493779725 s since 1904-01-01), "file name str"="D:\\Data\\Ultrasound\\LSCO\\LSCO22__130814c\\5_Cooling_2nd_try\\September_2014\\091714\\77.43400K_500_2500_2.10000V_0.00000T_Sep17-2014__02-22-05_001_091714.bin", "mod time(min)"=58229662.083333336, "file format"=enum."binary", "power(V)"=2.1, "Magn Field(T) "=0.0}, {"temperature"=77.354, "temperature str"="77.35400", "file path"=path "D:/Data/Ultrasound/LSCO/LSCO22__130814c/5_Cooling_2nd_try/September_2014/091714/77.35400K_500_2500_2.10000V_0.00000T_Sep17-2014__02-23-24_001_091714.bin", "last mod"=timestamp(3493779804 s since 1904-01-01), "file name str"="D:\\Data\\Ultrasound\\LSCO\\LSCO22__130814c\\5_Cooling_2nd_try\\September_2014\\091714\\77.35400K_500_2500_2.10000V_0.00000T_Sep17-2014__02-23-24_001_091714.bin", "mod time(min)"=58229663.4, "file format"=enum."binary", "power(V)"=2.1, "Magn Field(T) "=0.0}, {"temperature"=77.279, "temperature str"="77.27900", "file path"=path "D:/Data/Ultrasound/LSCO/LSCO22__130814c/5_Cooling_2nd_try/September_2014/091714/77.27900K_500_2500_2.10000V_0.00000T_Sep17-2014__02-24-44_001_091714.bin", "last mod"=timestamp(3493779884 s since 1904-01-01), "file name str"="D:\\Data\\Ultrasound\\LSCO\\LSCO22__130814c\\5_Cooling_2nd_try\\September_2014\\091714\\77.27900K_500_2500_2.10000V_0.00000T_Sep17-2014__02-24-44_001_091714.bin", 
